vi "getUpdates.vi"(8 "error in":errorcluster, 11 "Token":string) -> (0 "error out":errorcluster, 1 "ConnectionStatus":bool, 2 "UpdateUniversal":T1, 3 "Token":string)   [LabVIEW 2016]
uses:
  TypeDefs/UpdateUniversal.ctl
  TypeDefs/Method.ctl
  TypeDefs/QueryStringItems.ctl
  <vilib>/httpClient/LabVIEWHTTPClient.lvlib
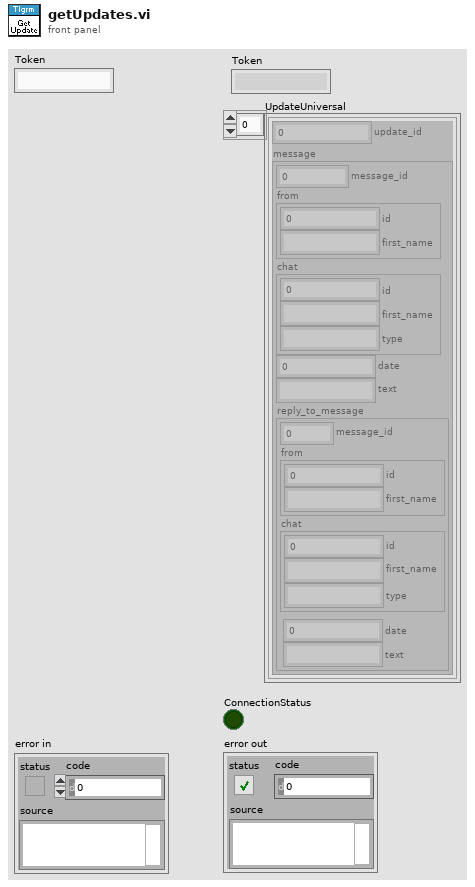
[diagram p1: front panel]
types:
  T1 = typedef "UpdateUniversal.ctl" = cluster{"update_id":u32, "message":cluster{"message_id":u32, "from":cluster{"id":u64, "first_name":string}, "chat":cluster{"id":i32, "first_name":string, "type":string}, "date":u32, "text":string, "reply_to_message":cluster{"message_id":u32, "from":cluster{"id":u64, "first_name":string}, "chat":cluster{"id":i32, "first_name":string, "type":string}, "date":u32, "text":string}}}[]
  T2 = typedef "QueryStringItems.ctl" = cluster{"QueryString":string, "QueryStringValue":string}[]
  T3 = typedef "Method.ctl" = string
  T4 = cluster{"QueryString":string, "QueryStringValue":string}
  T5 = cluster{"update_id":u32, "message":cluster{"message_id":u32, "from":cluster{"id":u64, "first_name":string}, "chat":cluster{"id":i32, "first_name":string, "type":string}, "date":u32, "text":string, "reply_to_message":cluster{"message_id":u32, "from":cluster{"id":u64, "first_name":string}, "chat":cluster{"id":i32, "first_name":string, "type":string}, "date":u32, "text":string}}}
  T6 = cluster{"QueryString":string, "QueryStringValue":string}[]
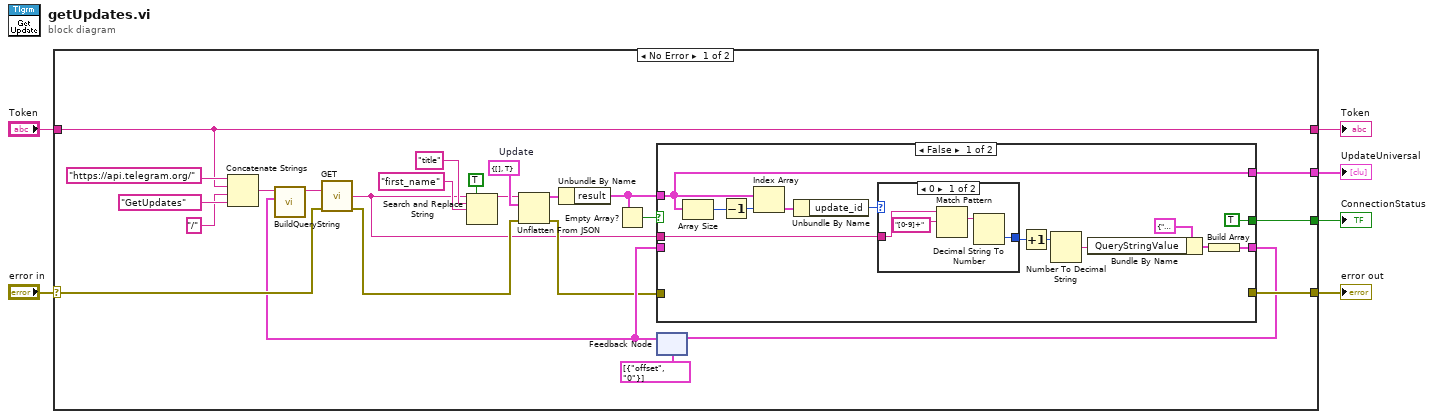
[diagram p0: block diagram]
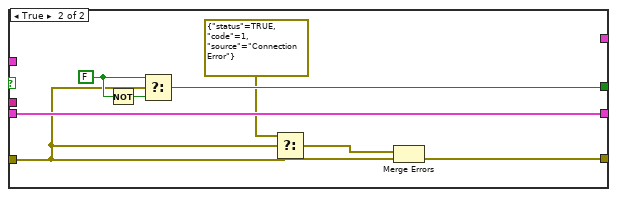
[diagram p3: hidden frame]
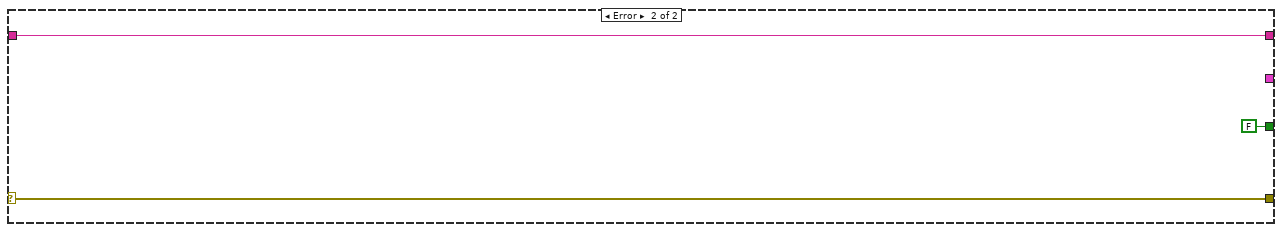
[diagram p4: hidden frame]
diagram:
  n1 = case shown="No Error" "error in" {
    selector: "error in" -> [w28 w59]
    tunnel: "Token" -> [w7 w57]
    tunnel: [w30 _] -> w6
    tunnel: [w29 w59] -> w5
    tunnel: [w27 FALSE ("status")] -> w1
    tunnel: [w7 w57] -> w2
    frame No Error {
      w24 = cluster{"result":T1, "ok":bool} {"result"=[], "ok"=TRUE}  # Update
      n2 = Concatenate Strings("https://api.telegram.org/" ("URL"), w7, "/" ("URL"), T3 "GetUpdates" ("Method")) -> (w13:string)
      n3 = feedback #1(T2 [{"QueryString"="offset", "QueryStringValue"="0"}] ("QueryStringItems")) -> (w26:T2)
      n4 = call "BuildQueryString.vi"("QueryStringItems"=w26, "QueryStringIn"=w13) -> ("QueryStringOut"=w14:string)  [unwired: 9 in]
      n5 = call <vilib>:"GET.vi"("url"=w14, "error in (no error)"=w28) -> ("body"=w10:string, "error out"=w19:errorcluster)  [unwired: 10 in, 2 out]
      n6 = Search and Replace String(replace all?=TRUE ("replace all? (F)"), input string=w10, search string="title" ("input string"), replace string="first_name" ("input string")) -> (result string=w20:string)  [unwired: 4 in, 3 out]
      n7 = Unflatten From JSON(JSON string=w20, type and defaults=w24, error in (no error)=w19) -> (value=w16:cluster{"result":T1, "ok":bool}, error out=w18:errorcluster)  [unwired: 4 in]
      n8 = Unbundle By Name(w16) -> ("result"=w17:T1)
      n9 = Empty Array?(array=w17) -> (empty?=w15:bool)
      n10 = case shown="False" w15 {
        tunnel: w17 -> [w35 _]
        tunnel: [w39 w56] -> w25
        tunnel: w26 -> [_ w56]
        tunnel: [w35 _] -> w30
        tunnel: w18 -> [_ w51]
        tunnel: [_ w55] -> w29
        tunnel: w10 -> [w36 _]
        tunnel: [TRUE ("status") w52] -> w27
        frame False {
          n11 = Array Size(array=w35) -> (size(s)=w42:i32)
          n12 = Decrement(x=w42) -> (x-1=w41:i32)
          n13 = Index Array(array=w35, index=w41) -> (element=w37:T5)
          n14 = Unbundle By Name(w37) -> ("update_id"=w38:u32)
          n15 = case shown="0" w38 {
            selector: w38 -> [_ w48]
            tunnel: w36 -> [w45 _]
            tunnel: [w44 w48] -> w32
            frame 0 {
              n16 = Match Pattern(string=w45, regular expression="[0-9]+") -> (match substring=w46:string)  [unwired: 1 in, 3 out]
              n17 = Decimal String To Number(string=w46) -> (number=w44:i32)  [unwired: 2 in, 1 out]
            }
            frame Default {
            }
          }
          n18 = Increment(x=w32) -> (x+1=w33:u32)
          n19 = Number To Decimal String(number=w33) -> (decimal integer string=w31:string)  [unwired: 1 in]
          n20 = Bundle By Name(cluster=T4 {"QueryString"="offset", "QueryStringValue"="0"} ("Cluster 2"), "QueryStringValue"=w31) -> (w40:T4)
          n21 = Build Array(w40) -> (w39:T6)
        }
        frame True {
          w53 = FALSE ("status")
          n22 = Not(x=w53) -> (.not. x?=w54:bool)
          n23 = Select(t=w53, s=w51, f=w54) -> (s? t:f=w52:bool)
          n24 = Select(t=errorcluster {"status"=TRUE, "code"=1, "source"="Connection Error"} ("error in"), s=w51, f=w51) -> (s? t:f=w49:errorcluster)
          n25 = Merge Errors(w49, w51) -> (w55:errorcluster)
        }
      }
      n26 = feedback-in #1(w25) -> ()
    }
    frame Error {
    }
  }
  "error out" <- w5
  "UpdateUniversal" <- w6
  "ConnectionStatus" <- w1
  "Token" <- w2
